vi "Get Execution Ref.vi"(8 "error in (no error)":errorcluster, 11 "Execution in":refnum<class "Execution.lvclass">) -> (0 "error out":errorcluster, 2 "Execution":refnum<k7>, 3 "Execution out":refnum<class "Execution.lvclass">)   [LabVIEW 2020, in "TSS.lvlib" / "Execution.lvclass"]
uses:
  Execution.lvclass
  Execution.lvclass/Execution.ctl
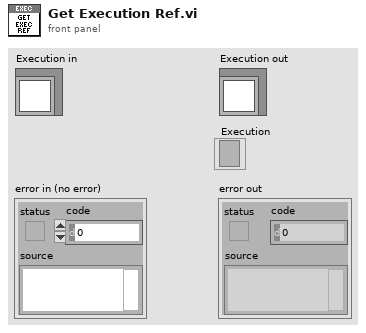
[diagram p1: front panel]
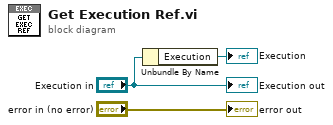
[diagram p0: block diagram]
diagram:
  n1 = Unbundle By Name("Execution in") -> ("Execution"=→"Execution":refnum<k7>)
  "error out" <- "error in (no error)"
  "Execution out" <- "Execution in"
